vi "Refactor Dependencies for VI.vi"(8 "error in (no error)":errorcluster, 10 "rename data":T3, 11 "vi path":path) -> (0 "error out":errorcluster, 1 "missing dependencies":bool, 2 "missing items":T2)   [LabVIEW 2020, in "MeasurementService Editor.lvlib"]
uses:
  MeasurementService Editor.lvlib
  Rename Refactor Data.ctl
  Rename Refactor Mapping Info.ctl
  Rename Refactor Result.ctl
  <vilib>/Utility/traverseref.llb/TRef TravTarget.ctl
  <vilib>/Utility/traverseref.llb/VI Scripting - Traverse.lvlib
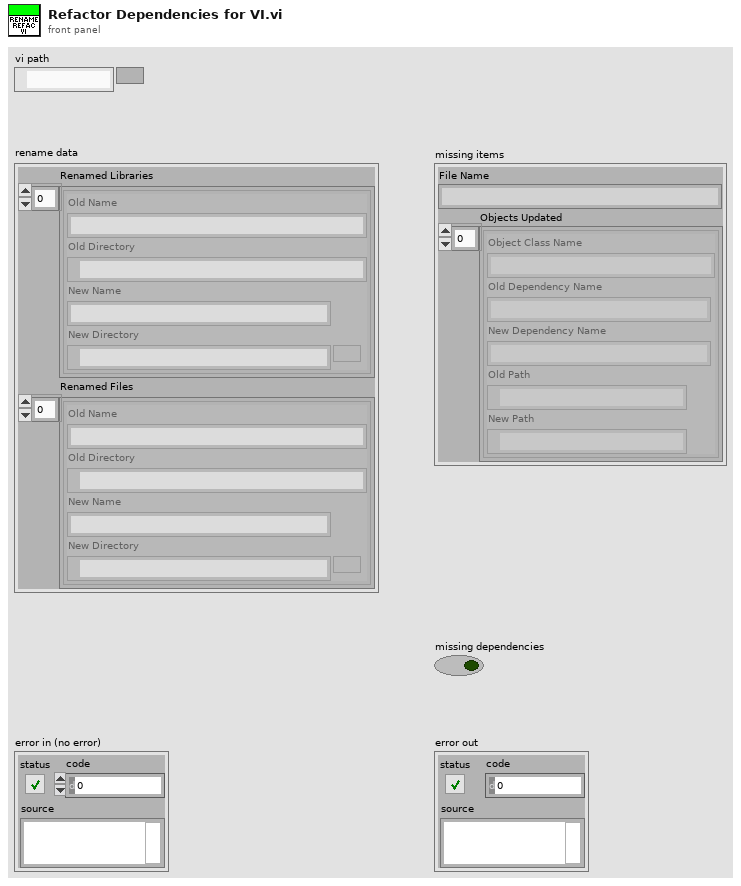
[diagram p1: front panel]
types:
  T1 = typedef "MeasurementService Editor.lvlib/Rename Refactor Result.ctl" = cluster{"Object Class Name":string, "Old Dependency Name":string, "New Dependency Name":string, "Old Path":path, "New Path":path}
  T2 = cluster{"File Name":string, "Objects Updated":T1[]}
  T3 = typedef "MeasurementService Editor.lvlib/Rename Refactor Data.ctl" = cluster{"Renamed Libraries":T4[], "Renamed Files":T4[]}
  T4 = typedef "MeasurementService Editor.lvlib/Rename Refactor Mapping Info.ctl" = cluster{"Old Name":string, "Old Directory":path, "New Name":string, "New Directory":path}
  T5 = typedef "TRef TravTarget.ctl" = enum16{"FP", "BD", "Other"}
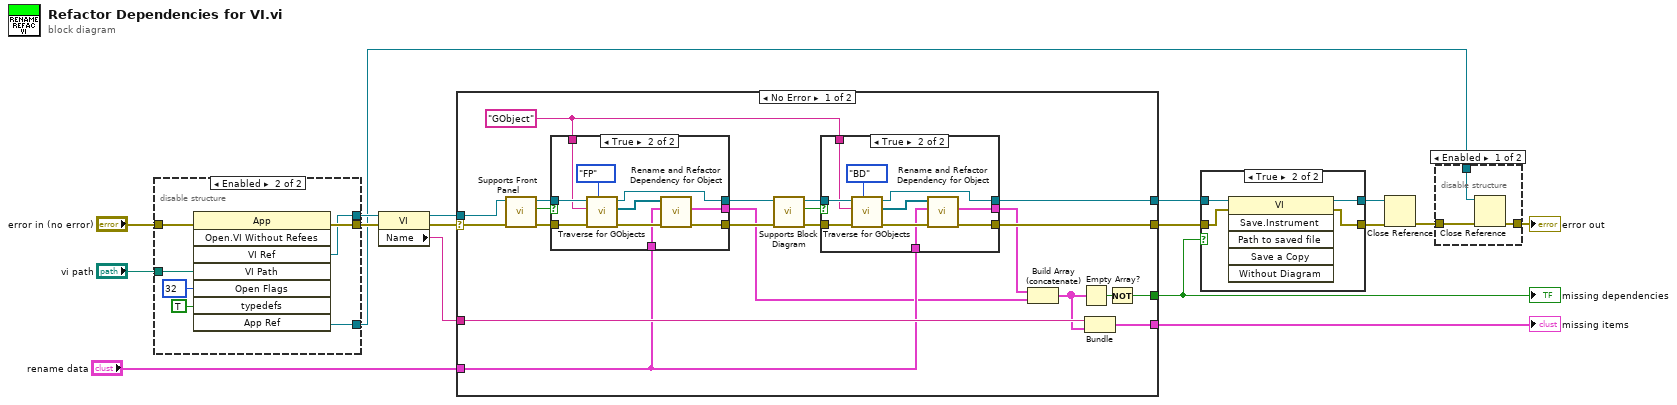
[diagram p0: block diagram]
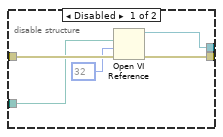
[diagram p4: hidden frame]
diagram:
  n1 = disable-structure shown="Enabled" {
    disable-tunnel: [w22 w25] -> w17
    disable-tunnel: "error in (no error)" -> [w21 w28]
    disable-tunnel: "vi path" -> [w20 w26]
    disable-tunnel: [w19 w27] -> w14
    disable-tunnel: [_ w24] -> w8
    frame Disabled {
      n2 = Open VI Reference(vi path=w20, options=32, error in (no error)=w21) -> (vi reference=w22:refnum<vi>, error out=w19:errorcluster)  [unwired: 3 in]
    }
    frame Enabled {
      n3 = invoke class="App" method="Open.VI Without Refees"(error in=w28, "VI Path"=w26, "Open Flags"=32 ("options"), "typedefs"=TRUE ("Load Typedefs?")) -> (error out=w27:errorcluster, "VI Ref"=w25:refnum<vi>, "App Ref"=w24:refnum<vi>)  [unwired: 4 in, 5 out]
    }
  }
  n4 = property class="VI"(reference=w17, error in=w14) -> (reference out=w12:refnum<vi>, error out=w11:errorcluster, "Name"=w13:string)
  n5 = case shown="No Error" w11 {
    selector: w11 -> [w46 w76]
    tunnel: [w50 _] -> w5
    tunnel: [w49 _] -> w6
    tunnel: w13 -> [w48 _]
    tunnel: w12 -> [w47 w75]
    tunnel: [w45 w76] -> w4
    tunnel: [w44 w75] -> w2
    tunnel: "rename data" -> [w32 _]
    frame No Error {
      w42 = "GObject" ("Class Name")
      n6 = call "Supports Front Panel.vi"("error in (no error)"=w46, "vi in"=w47) -> ("error out"=w38:errorcluster, "has front panel"=w39:bool, "vi out"=w40:refnum<vi>)  [unwired: 7 in]
      n7 = case shown="True" w39 {
        tunnel: w40 -> [w64 w72]
        tunnel: [w64 w65] -> w36
        tunnel: [w63 w71] -> w37
        tunnel: w42 -> [_ w70]
        tunnel: [_ w69] -> w30
        tunnel: w38 -> [w63 w68]
        tunnel: w32 -> [_ w66]
        frame False {
          # "poly VIs don't have front panels"
        }
        frame True {
          n8 = call <vilib>:"Traverse for GObjects.vi"("Traverse Target"=TRef_TravTarget."FP", "error in (no error)"=w68, "Class Name"=w70, "VI Refnum"=w72) -> ("error out"=w74:errorcluster, "References"=w67:refnum<vi>[], "dup VI Refnum"=w65:refnum<vi>)  [unwired: 4 in, 1 out]
          n9 = call "Rename and Refactor Dependency for Object.vi"("error in (no error)"=w74, "rename data"=w66, "object references"=w67) -> ("error out"=w71:errorcluster, "refactor results"=w69:T1[])  [unwired: 7 in]
        }
      }
      n10 = call "Supports Block Diagram.vi"("error in (no error)"=w37, "vi in"=w36) -> ("error out"=w33:errorcluster, "has block diagram"=w34:bool, "vi out"=w35:refnum<vi>)  [unwired: 7 in]
      n11 = case shown="True" w34 {
        tunnel: w35 -> [w51 w61]
        tunnel: w42 -> [_ w60]
        tunnel: [w52 w55] -> w45
        tunnel: [w51 w54] -> w44
        tunnel: w33 -> [w52 w59]
        tunnel: w32 -> [_ w56]
        tunnel: [_ w53] -> w31
        frame False {
        }
        frame True {
          n12 = call <vilib>:"Traverse for GObjects.vi"("Traverse Target"=TRef_TravTarget."BD", "error in (no error)"=w59, "Class Name"=w60, "VI Refnum"=w61) -> ("error out"=w58:errorcluster, "References"=w57:refnum<vi>[], "dup VI Refnum"=w54:refnum<vi>)  [unwired: 4 in, 1 out]
          n13 = call "Rename and Refactor Dependency for Object.vi"("error in (no error)"=w58, "rename data"=w56, "object references"=w57) -> ("error out"=w55:errorcluster, "refactor results"=w53:T1[])  [unwired: 7 in]
        }
      }
      n14 = Build Array (concatenate)(w31, w30) -> (w41:T1[])
      n15 = Empty Array?(array=w41) -> (empty?=w43:bool)
      n16 = Bundle("Name"=w48, w41) -> (w49:cluster{"Name":string, T1[]})  [unwired: 1 in]
      n17 = Not(x=w43) -> (.not. x?=w50:bool)
    }
    frame Error {
    }
  }
  "missing dependencies" <- w5
  "missing items" <- w6
  n18 = case shown="True" w5 {
    tunnel: w4 -> [w78 w81]
    tunnel: [w78 w79] -> w3
    tunnel: w2 -> [w77 w82]
    tunnel: [w77 w80] -> w1
    frame False {
    }
    frame True {
      n19 = invoke class="VI" method="Save.Instrument"(reference=w82, error in=w81) -> (reference out=w80:refnum<vi>, error out=w79:errorcluster)  [unwired: 4 in, 4 out]
    }
  }
  n20 = Close Reference(reference=w1, error in (no error)=w3) -> (error out=w10:errorcluster)
  n21 = disable-structure shown="Enabled" {
    disable-tunnel: w10 -> [w85 w86]
    disable-tunnel: [w84 w86] -> w9
    disable-tunnel: w8 -> [w83 _]
    frame Enabled {
      n22 = Close Reference(reference=w83, error in (no error)=w85) -> (error out=w84:errorcluster)
    }
    frame Disabled {
    }
  }
  "error out" <- w9
